vi "Create Tolerancing Bundles.vi"(9 "Channel Description":string[][](array[string]), 11 "Machine Specifications":string[][](array[string])) -> (3 "Tolerancing Bundle":T1(array[cluster]))   [LabVIEW 2013]
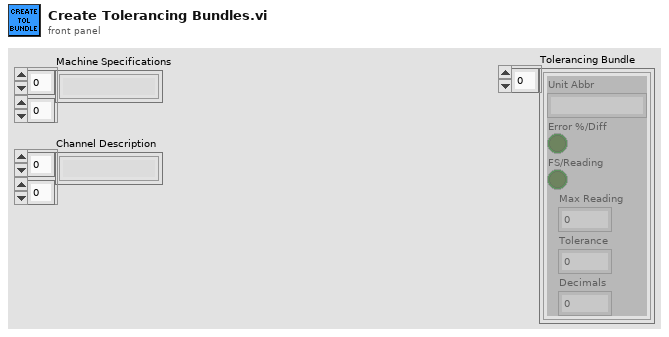
[diagram p1: front panel]
types:
  T1 = cluster{"Unit Abbr":string, "Error %/Diff":bool, "FS/Reading":bool, "Max Reading":dbl, "Tolerance":dbl, "Decimals":i16}[]
  T2 = cluster{"Unit Abbr":string, "Error %/Diff":bool, "FS/Reading":bool, "Max Reading":dbl, "Tolerance":dbl, "Decimals":i16}
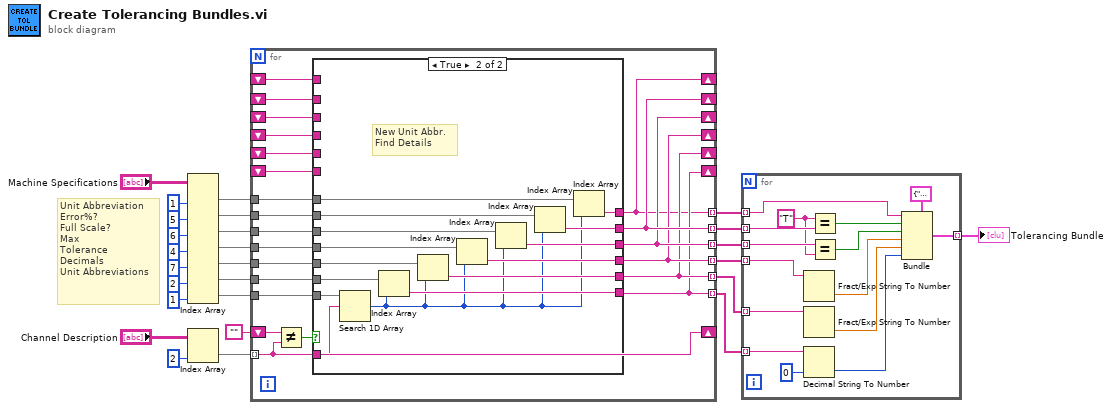
[diagram p0: block diagram]
diagram:
  # "Unit Abbreviation\nError%?\nFull Scale?\nMax\nTolerance\nDecimals\nUnit Abbreviations"
  n1 = Index Array(array="Machine Specifications", index (col) #1=1 ("disabled index (col)"), index (col) #2=5 ("disabled index (col)"), index (col) #3=6 ("index (col)"), index (col) #4=4 ("index (col)"), index (col) #5=7 ("index (col)"), index (col) #6=2 ("index (col)"), index (col) #7=1 ("index (col)")) -> (element #1=w21:string[], element #2=w6:string[], element #3=w5:string[], element #4=w4:string[], element #5=w3:string[], element #6=w18:string[], element #7=w19:string[])  [unwired: 7 in]
  n2 = Index Array(array="Channel Description", index (col)=2 ("disabled index (col)")) -> (element=w12:string[])  [unwired: 1 in]
  n3 = for {
    tunnel: w12 -> [w27] mode=indexing
    tunnel: w6 -> [w43]
    tunnel: w5 -> [w44]
    tunnel: w4 -> [w45]
    tunnel: w3 -> [w46]
    tunnel: [w42] -> w26 mode=indexing
    tunnel: [w41] -> w25 mode=indexing
    tunnel: [w40] -> w24 mode=indexing
    shift-right: [w42] -> _
    shift-left: _ -> [w37]
    shift-right: [w41] -> _
    shift-left: _ -> [w38]
    shift-right: [w40] -> _
    shift-left: _ -> [w39]
    tunnel: w18 -> [w35]
    tunnel: w19 -> [w36]
    tunnel: [w33] -> w22 mode=indexing
    tunnel: [w34] -> w23 mode=indexing
    shift-right: [w34] -> _
    shift-left: _ -> [w32]
    shift-right: [w33] -> _
    shift-left: _ -> [w31]
    tunnel: w21 -> [w30]
    shift-right: [w28] -> _
    shift-left: _ -> [w29]
    tunnel: [w28] -> w2 mode=indexing
    shift-right: [w27] -> _
    shift-left: "" -> [w48]
    n4 = Not Equal?(x=w48, y=w27) -> (x != y?=w47:bool)
    n5 = case shown="True" w47 {
      tunnel: w27 -> [_ w69]
      tunnel: w46 -> [_ w61]
      tunnel: w45 -> [_ w68]
      tunnel: w44 -> [_ w67]
      tunnel: w43 -> [_ w66]
      tunnel: [w54 w65] -> w42
      tunnel: [w53 w64] -> w41
      tunnel: [w52 w63] -> w40
      tunnel: w39 -> [w52 _]
      tunnel: w38 -> [w53 _]
      tunnel: w37 -> [w54 _]
      tunnel: w36 -> [_ w62]
      tunnel: w35 -> [_ w60]
      tunnel: [w50 w59] -> w33
      tunnel: [w51 w58] -> w34
      tunnel: w32 -> [w51 _]
      tunnel: w31 -> [w50 _]
      tunnel: w30 -> [_ w57]
      tunnel: [w49 w55] -> w28
      tunnel: w29 -> [w49 _]
      frame False {
        # "Same Unit Abbr.\nUse previous\navoid searching"
      }
      frame True {
        # "New Unit Abbr.\nFind Details"
        n6 = Search 1D Array(1D array=w62, element=w69) -> (index of element=w56:i32)  [unwired: 1 in]
        n7 = Index Array(array=w60, index=w56) -> (element=w59:string)
        n8 = Index Array(array=w61, index=w56) -> (element=w58:string)
        n9 = Index Array(array=w68, index=w56) -> (element=w63:string)
        n10 = Index Array(array=w67, index=w56) -> (element=w64:string)
        n11 = Index Array(array=w66, index=w56) -> (element=w65:string)
        n12 = Index Array(array=w57, index=w56) -> (element=w55:string)
      }
    }
  }
  n13 = for {
    tunnel: w26 -> [w83] mode=indexing
    tunnel: w25 -> [w84] mode=indexing
    tunnel: w24 -> [w81] mode=indexing
    tunnel: w23 -> [w80] mode=indexing
    tunnel: w22 -> [w79] mode=indexing
    tunnel: w2 -> [w71] mode=indexing
    tunnel: [w70] -> w1 mode=indexing
    w82 = "T"
    n14 = Fract/Exp String To Number(string=w81) -> (number=w74:dbl)  [unwired: 3 in, 1 out]
    n15 = Fract/Exp String To Number(string=w80) -> (number=w75:dbl)  [unwired: 3 in, 1 out]
    n16 = Decimal String To Number(string=w79, default (0L)=i16 0) -> (number=w76:i16)  [unwired: 1 in, 1 out]
    n17 = Equal?(x=w82, y=w83) -> (x = y?=w72:bool)
    n18 = Equal?(x=w84, y=w82) -> (x = y?=w73:bool)
    n19 = Bundle(cluster=T2 {"Unit Abbr"="", "Error %/Diff"=FALSE, "FS/Reading"=FALSE, "Max Reading"=0.0, "Tolerance"=0.0, "Decimals"=0}, "Unit Abbr"=w71, "Error %/Diff"=w72, "FS/Reading"=w73, "Max Reading"=w74, "Tolerance"=w75, "Decimals"=w76) -> (w70:T2)
  }
  "Tolerancing Bundle" <- w1
